vi "Execute.vi"(8 "error in (no error)":errorcluster, 9 "Workspace":T1, 10 "Cluster":T2, 11 "Pick and Place in":refnum<class "Pick and Place.lvclass">) -> (0 "error out":errorcluster, 2 "Control Out":T2, 3 "Pick and Place out":refnum<class "Pick and Place.lvclass">)   [LabVIEW 2019, in "Pick and Place.lvclass"]
uses:
  Pick and Place.lvclass
  Controller/Controllers.ctl
  Controller/I-O/I-O.lvclass
  Controller/Dispenser/Dispenser.lvclass
  C:/Program Files (x86)/Aerotech/A3200/LabVIEW/2010/Bin/Aerotech.A3200.dll
  Program Files (x86)/Aerotech/A3200/LabVIEW/2010/Bin/Aerotech.A3200.dll
  Workspace/Workspace.ctl
  Pick and Place.lvclass/Pick and Place.ctl
  1ece5d4e-95c1-4e54-a598-3678f2710534.vi
  Controller/Motion/A3200/A3200.lvclass
  Controller/Controller.lvclass
  Workspace/Fixture.lvclass
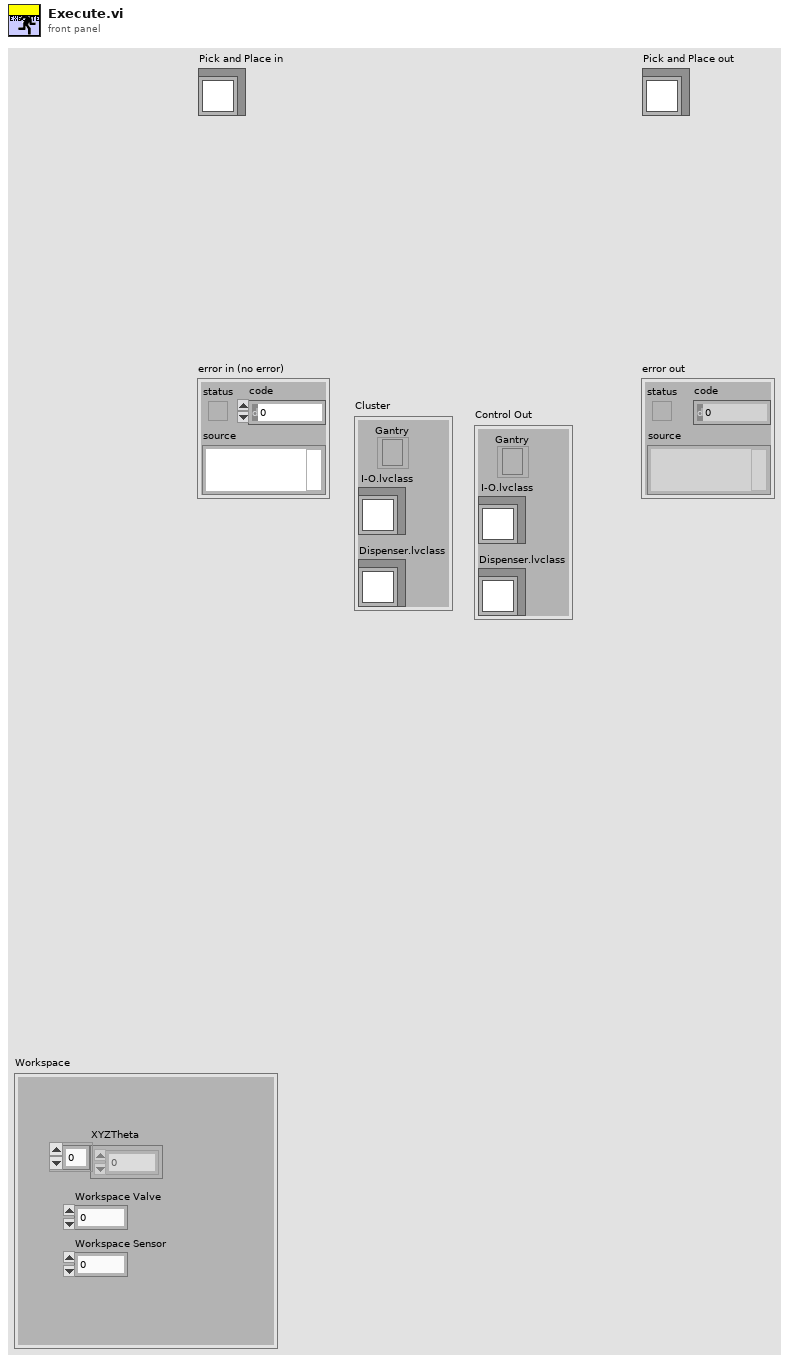
[diagram p1: front panel]
types:
  T1 = typedef "Fixture.lvclass/Workspace.ctl" = cluster{"XYZTheta":dbl[], "Workspace Valve":i32, "Workspace Sensor":i32}
  T2 = typedef "Controller.lvclass/Controllers.ctl" = cluster{"I-O.lvclass":refnum<class "I-O.lvclass">, "Dispenser.lvclass":refnum<class "Dispenser.lvclass">, "Gantry":refnum<k24>}
  T3 = typedef "Pick and Place.lvclass/Pick and Place Type.ctl" = enum16{"Primary Pick Up", "Secondary Pick Up", "Put Down All", "Pick Up All", "Put Down Secondary"}
  T4 = typedef "I-O.lvclass/Pin Map.ctl" = cluster{"Region Valves":i32[], "Extra Valves":dbl[][][], "Tool Primary Valve":i32, "Tool Secondary Valve":i32, "Region Sensors":i32[], "Extra Sensors":dbl[][][], "Tool Primary Sensor":dbl, "Tool Secondary Sensor":dbl, "Compression Sensor":dbl, "5V":i32}
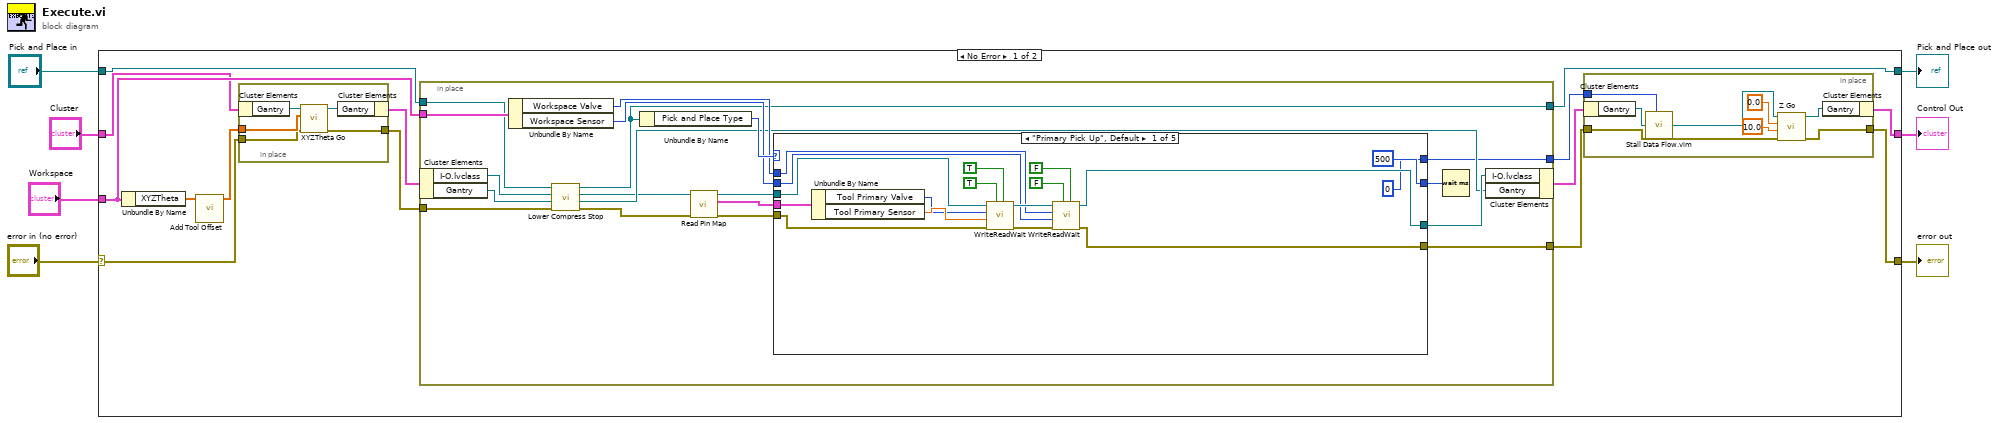
[diagram p0: block diagram]
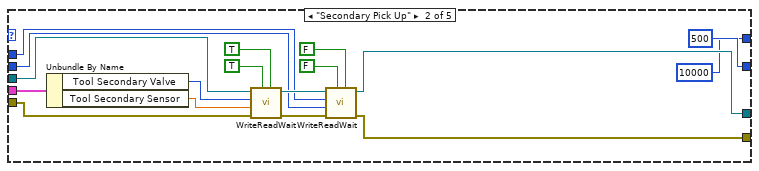
[diagram p2: hidden frame]
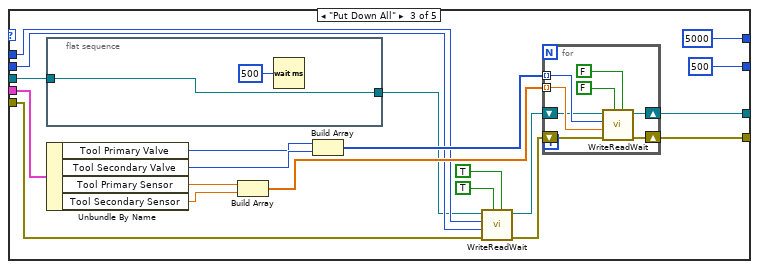
[diagram p3: hidden frame]
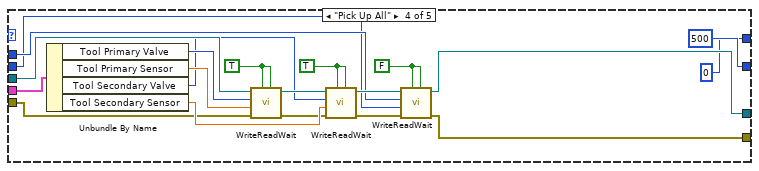
[diagram p4: hidden frame]
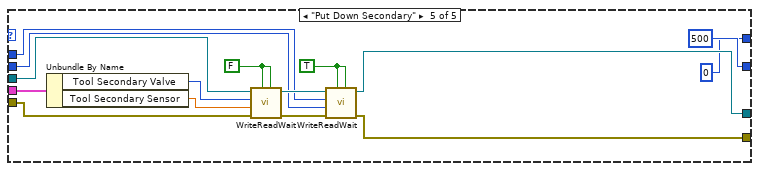
[diagram p5: hidden frame]
diagram:
  n1 = case shown="No Error" "error in (no error)" {
    selector: "error in (no error)" -> [w12 w154]
    tunnel: "Cluster" -> [w18 w155]
    tunnel: "Workspace" -> [w19 _]
    tunnel: [w8 w154] -> w1
    tunnel: [w17 w155] -> w2
    tunnel: "Pick and Place in" -> [w16 w153]
    tunnel: [w15 w153] -> w6
    frame No Error {
      n2 = Unbundle By Name(w19) -> ("XYZTheta"=w14:dbl[])
      n3 = call "Add Tool Offset.vi"("XYZTheta"=w14) -> ("Array"=w13:dbl[])  [unwired: 10 in]
      n4 = in-place {
        in-place-border: w13 -> [w152]
        in-place-border: w12 -> [w149]
        in-place-border: [w148] -> w11
        n5 = in-place-cluster #1(w18) -> ("Gantry"=w151:refnum<k24>)
        n6 = call "XYZTheta Go.vi"("error in (no error)"=w149, "XYZTheta In"=w152, "Gantry In"=w151) -> ("error out"=w148:errorcluster, "Gantry Out"=w150:refnum<k24>)  [unwired: 6 in, 1 out]
        n7 = in-place-cluster #1("Gantry"=w150) -> (w21:T2)
      }
      n8 = in-place {
        in-place-border: w19 -> [w40]
        in-place-border: w16 -> [w28]
        in-place-border: [w27] -> w15
        in-place-border: w11 -> [w26]
        in-place-border: [w23] -> w10
        in-place-border: [w22] -> w9
        n9 = in-place-cluster #2(w21) -> ("I-O.lvclass"=w33:refnum<class "I-O.lvclass">, "Gantry"=w32:refnum<k24>)
        n10 = Unbundle By Name(w40) -> ("Workspace Valve"=w38:i32, "Workspace Sensor"=w37:i32)
        n11 = call "Lower Compress Stop.vi"("error in (no error)"=w26, "Gantry In"=w32, "I-O.lvclass"=w33, "Pick and Place in"=w28) -> ("error out"=w25:errorcluster, "Gantry Out"=w30:refnum<k24>, "I-O out"=w29:refnum<class "I-O.lvclass">, "Pick and Place Out"=w27:refnum<class "Pick and Place.lvclass">)  [unwired: 4 in]
        n12 = Unbundle By Name(w27) -> ("Pick and Place Type"=w39:T3)
        n13 = call-dynamic "Read Pin Map.vi"("error in (no error)"=w25, "I-O in"=w29) -> ("error out"=w24:errorcluster, "Pin Map 2"=w35:T4, "I-O out"=w34:refnum<class "I-O.lvclass">)  [unwired: 7 in]
        n14 = case shown="\"Primary Pick Up\", Default" w39 {
          tunnel: w38 -> [w54 w66 w84 w114 w133]
          tunnel: w37 -> [w53 w65 w83 w113 w132]
          tunnel: [w48 w64 w88 w111 w130] -> w31
          tunnel: [u32 500 ("milliseconds to wait") 500 500 u32 500 ("milliseconds to wait") u32 500 ("milliseconds to wait")] -> w36
          tunnel: w34 -> [w47 w63 w79 w123 w138]
          tunnel: w35 -> [w46 w62 w82 w124 w139]
          tunnel: w24 -> [w44 w61 w78 w109 w128]
          tunnel: [w42 w59 w76 w106 w126] -> w23
          tunnel: [u32 0 ("milliseconds to wait") u32 10000 ("milliseconds to wait") u32 5000 ("milliseconds to wait") u32 0 ("milliseconds to wait") u32 0 ("milliseconds to wait")] -> w22
          frame "Primary Pick Up", Default {
            n15 = Unbundle By Name(w46) -> ("Tool Primary Valve"=w45:i32, "Tool Primary Sensor"=w56:dbl)
            n16 = call "WriteReadWait.vi"("Read Value"=TRUE, "Write Value"=TRUE, "error in (no error)"=w44, "Read"=w56, "Write"=w45, "I-O in"=w47) -> ("error out"=w43:errorcluster, "I-O out"=w55:refnum<class "I-O.lvclass">)  [unwired: 4 in]
            n17 = call "WriteReadWait.vi"("Read Value"=FALSE ("Write Value"), "Write Value"=FALSE ("Read Value"), "error in (no error)"=w43, "Read"=w53, "Write"=w54, "I-O in"=w55) -> ("error out"=w42:errorcluster, "I-O out"=w48:refnum<class "I-O.lvclass">)  [unwired: 4 in]
          }
          frame "Secondary Pick Up" {
            n18 = Unbundle By Name(w62) -> ("Tool Secondary Valve"=w68:i32, "Tool Secondary Sensor"=w67:dbl)
            n19 = call "WriteReadWait.vi"("Read Value"=TRUE, "Write Value"=TRUE, "error in (no error)"=w61, "Read"=w67, "Write"=w68, "I-O in"=w63) -> ("error out"=w60:errorcluster, "I-O out"=w73:refnum<class "I-O.lvclass">)  [unwired: 4 in]
            n20 = call "WriteReadWait.vi"("Read Value"=FALSE ("Write Value"), "Write Value"=FALSE ("Read Value"), "error in (no error)"=w60, "Read"=w65, "Write"=w66, "I-O in"=w73) -> ("error out"=w59:errorcluster, "I-O out"=w64:refnum<class "I-O.lvclass">)  [unwired: 4 in]
          }
          frame "Put Down All" {
            n21 = flat-sequence {
              tunnel: [w95] -> w80
              tunnel: w79 -> [w95]
              frame #0 {
                # "Delay After Placing"
                n22 = Wait (ms)(milliseconds to wait=u32 500) -> ()  [unwired: 1 out]
              }
            }
            n23 = Unbundle By Name(w82) -> ("Tool Primary Valve"=w89:i32, "Tool Secondary Valve"=w90:i32, "Tool Primary Sensor"=w91:dbl, "Tool Secondary Sensor"=w92:dbl)
            n24 = Build Array(w91, w92) -> (w94:dbl[])
            n25 = Build Array(w89, w90) -> (w93:i32[])
            n26 = call "WriteReadWait.vi"("Read Value"=TRUE, "Write Value"=TRUE, "error in (no error)"=w78, "Read"=w83, "Write"=w84, "I-O in"=w80) -> ("error out"=w77:errorcluster, "I-O out"=w81:refnum<class "I-O.lvclass">)  [unwired: 4 in]
            n27 = for {
              shift-right: [w99] -> w88
              shift-left: w81 -> [w100]
              tunnel: w93 -> [w102] mode=indexing
              tunnel: w94 -> [w101] mode=indexing
              shift-right: [w97] -> w76
              shift-left: w77 -> [w98]
              n28 = call "WriteReadWait.vi"("Read Value"=FALSE ("Write Value"), "Write Value"=FALSE ("Read Value"), "error in (no error)"=w98, "Read"=w101, "Write"=w102, "I-O in"=w100) -> ("error out"=w97:errorcluster, "I-O out"=w99:refnum<class "I-O.lvclass">)  [unwired: 4 in]
            }
          }
          frame "Pick Up All" {
            w112 = FALSE ("Read Value")
            w116 = TRUE ("Write Value")
            w122 = TRUE ("Write Value")
            n29 = Unbundle By Name(w124) -> ("Tool Primary Valve"=w121:i32, "Tool Primary Sensor"=w120:dbl, "Tool Secondary Valve"=w118:i32, "Tool Secondary Sensor"=w117:dbl)
            n30 = call "WriteReadWait.vi"("Read Value"=w122, "Write Value"=w122, "error in (no error)"=w109, "Read"=w120, "Write"=w121, "I-O in"=w123) -> ("error out"=w108:errorcluster, "I-O out"=w119:refnum<class "I-O.lvclass">)  [unwired: 4 in]
            n31 = call "WriteReadWait.vi"("Read Value"=w116, "Write Value"=w116, "error in (no error)"=w108, "Read"=w117, "Write"=w118, "I-O in"=w119) -> ("error out"=w107:errorcluster, "I-O out"=w115:refnum<class "I-O.lvclass">)  [unwired: 4 in]
            n32 = call "WriteReadWait.vi"("Read Value"=w112, "Write Value"=w112, "error in (no error)"=w107, "Read"=w113, "Write"=w114, "I-O in"=w115) -> ("error out"=w106:errorcluster, "I-O out"=w111:refnum<class "I-O.lvclass">)  [unwired: 4 in]
          }
          frame "Put Down Secondary" {
            w131 = TRUE ("Read Value")
            w135 = FALSE ("Write Value")
            n33 = Unbundle By Name(w139) -> ("Tool Secondary Valve"=w137:i32, "Tool Secondary Sensor"=w136:dbl)
            n34 = call "WriteReadWait.vi"("Read Value"=w135, "Write Value"=w135, "error in (no error)"=w128, "Read"=w136, "Write"=w137, "I-O in"=w138) -> ("error out"=w127:errorcluster, "I-O out"=w134:refnum<class "I-O.lvclass">)  [unwired: 4 in]
            n35 = call "WriteReadWait.vi"("Read Value"=w131, "Write Value"=w131, "error in (no error)"=w127, "Read"=w132, "Write"=w133, "I-O in"=w134) -> ("error out"=w126:errorcluster, "I-O out"=w130:refnum<class "I-O.lvclass">)  [unwired: 4 in]
          }
        }
        n36 = Wait (ms)(milliseconds to wait=w36) -> ()  [unwired: 1 out]
        n37 = in-place-cluster #2("I-O.lvclass"=w31, "Gantry"=w30) -> (w20:T2)
      }
      n38 = in-place {
        in-place-border: w10 -> [w142]
        in-place-border: w9 -> [w146]
        in-place-border: [w143] -> w8
        n39 = in-place-cluster #3(w20) -> ("Gantry"=w147:refnum<k24>)
        n40 = call "Stall Data Flow.vim"("value in"=w147, "milliseconds to wait"=w146) -> ("value out"=w145:refnum<k24>)  [unwired: 1 out]
        n41 = call "Z Go.vi"("error in (no error)"=w142, "Speed"=10.0, "Position"=0.0, "Gantry In"=w145) -> ("error out"=w143:errorcluster, "Gantry Out"=w144:refnum<k24>)  [unwired: 6 in]
        n42 = in-place-cluster #3("Gantry"=w144) -> (w17:T2)
      }
    }
    frame Error {
    }
  }
  "error out" <- w1
  "Pick and Place out" <- w6
  "Control Out" <- w2
